vi "Speed Transform with Accel.vi"(8 "Reset Encoder 0":bool, 9 "w":dbl(slide) scale=-5.0..5.0, 10 "Vy":dbl(slide) scale=-1.0..1.0, 11 "Vx":dbl(slide) scale=-1.0..1.0) -> (3 "Distance & Speed Cluster":T1)   [LabVIEW 2018]
panel:
  in  "stop":bool
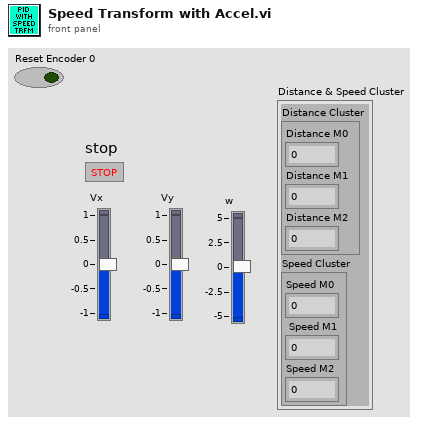
[diagram p1: front panel]
types:
  T1 = cluster{"Distance Cluster":cluster{"Distance M0 ":dbl, "Distance M1 ":dbl, "Distance M2 ":dbl}, "Speed Cluster":cluster{"Speed M0":dbl, " Speed M1":dbl, "Speed M2":dbl}}
  T2 = cluster{"Speed M0":dbl, " Speed M1":dbl, "Speed M2":dbl}
  T3 = cluster{"Distance M0 ":dbl, "Distance M1 ":dbl, "Distance M2 ":dbl}
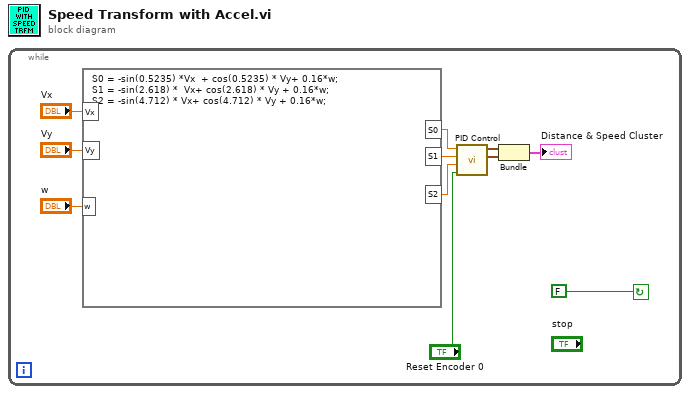
[diagram p0: block diagram]
diagram:
  n1 = while {
    stop <- FALSE ("Boolean") continue-if-true
    n2 = formula code="S0 = -sin(0.5235) *Vx  + cos(0.5235) * Vy+ 0.16*w;\nS1 = -sin(2.618) *  Vx+ cos(2.618) * Vy + 0.16*w;\nS2 = -sin(4.712) * Vx+ cos(4.712) * Vy + 0.16*w;"("Vx"="Vx", "Vy"="Vy", "w"="w") -> ("S0"=w11:dbl, "S1"=w10:dbl, "S2"=w9:dbl)
    n3 = call "PID Control.vi"("Reset Encoder 0"="Reset Encoder 0", "M2 Setpoint"=w9, "M1 Setpoint"=w10, "M0 Setpoint"=w11) -> ("Speed Cluster"=w4:T2, "Distance Cluster"=w5:T3)  [unwired: 6 in]
    n4 = Bundle("Distance Cluster"=w5, "Speed Cluster"=w4) -> (→"Distance & Speed Cluster":T1)  [unwired: 1 in]
  }
